vi "Process Session Status.vi"(8 "error in (no error)":errorcluster, 11 "session ID in":i32 format="%.0x") -> (0 "error out":errorcluster, 1 "stderr":string, 2 "stdout":string, 3 "session ID out":i32 format="%.0x", 4 "running":bool)   [LabVIEW 2013]
uses:
  ProcessSession.dll
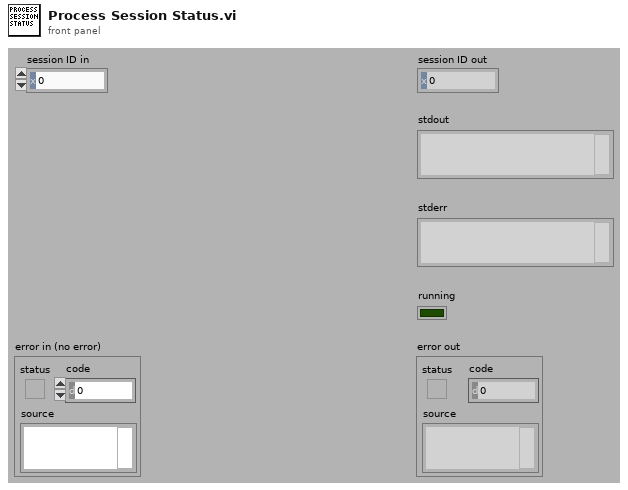
[diagram p1: front panel]
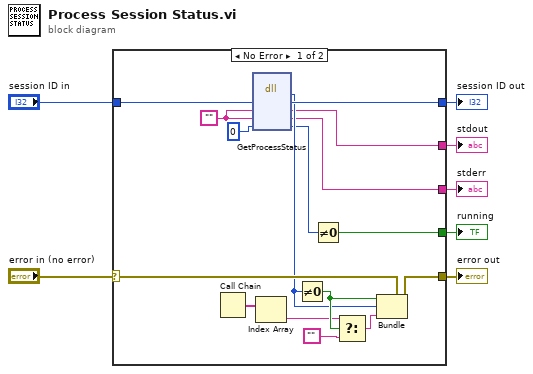
[diagram p0: block diagram]
diagram:
  n1 = case shown="No Error" "error in (no error)" {
    selector: "error in (no error)" -> [w23 w25]
    tunnel: [w16 w24] -> w7
    tunnel: [w19 w25] -> w5
    tunnel: [w11 _] -> w4
    tunnel: [w10 _] -> w3
    tunnel: [w9 _] -> w2
    tunnel: "session ID in" -> [w8 w24]
    frame No Error {
      w14 = ""
      n2 = Call Chain() -> (call chain=w18:string[])
      n3 = dll-call lib="C:/Users/inghoshr/Documents/LabVIEW Data/SmoketestVMVi/Process Session/ProcessSession.dll" fn="GetProcessStatus"("session"=w8, "stdoutData"=w14, "stderrData"=w14, "stillRunning"=0) -> (w15:i32, "session"=w16:i32, "stdoutData"=w11:string, "stderrData"=w10:string, "stillRunning"=w12:i32)  [unwired: 3 in, 2 out]
      n4 = Index Array(array=w18) -> (element=w17:string)  [unwired: 1 in]
      n5 = Not Equal To 0?(x=w15) -> (x != 0?=w22:bool)
      n6 = Not Equal To 0?(x=w12) -> (x != 0?=w9:bool)
      n7 = Select(t=w17, s=w22, f="") -> (s? t:f=w20:string)
      n8 = Bundle(cluster=w23, "status"=w22, "code"=w15, "source"=w20) -> (w19:errorcluster)
    }
    frame Error {
    }
  }
  "session ID out" <- w7
  "error out" <- w5
  "stderr" <- w3
  "running" <- w2
  "stdout" <- w4
